vi "intrinsicfilestring.vi"(9 "Postfix":string=".tiff", 10 "Frame number":dbl, 11 "Trigger number":dbl) -> (3 "Filestring":string)   [LabVIEW 2016]
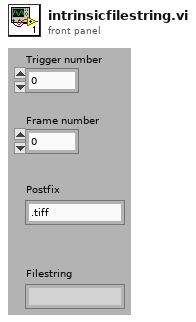
[diagram p1: front panel]
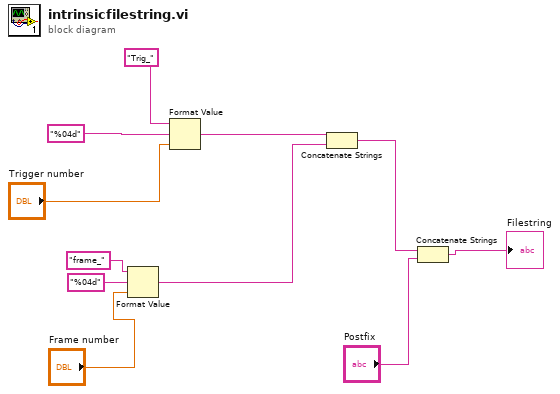
[diagram p0: block diagram]
diagram:
  n1 = Format Value(string ("")="frame_", format string="%04d", value (0)="Frame number") -> (output string=w3:string)
  n2 = Format Value(string ("")="Trig_", format string="%04d", value (0)="Trigger number") -> (output string=w4:string)
  n3 = Concatenate Strings(w4, w3) -> (w2:string)
  n4 = Concatenate Strings(w2, "Postfix") -> (→"Filestring":string)
